vi "EVT Camera Get Value Enum Param.vi"(9 "value":u32, 10 "name":string, 11 "camera":u64) -> (1 "value out":u32, 3 "function return":u32(ring))   [LabVIEW 2019, in "EmergentCameraC.lvlib"]
doc: "EMERGENTCAMERAC_API EVT_ERROR EVT_CameraGetValueEnumParam(Camera_Handle camera, const char* name, unsigned int* value);"
uses:
  EmergentCameraC.lvlib
  emergentInstall_Windows/win64/eSDK/bin/EmergentCameraC.dll
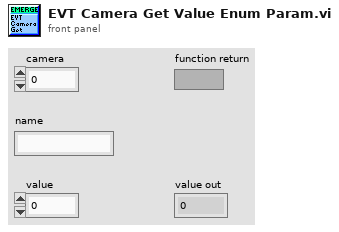
[diagram p1: front panel]
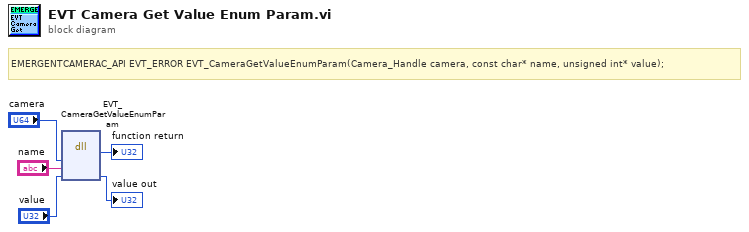
[diagram p0: block diagram]
diagram:
  # "EMERGENTCAMERAC_API EVT_ERROR EVT_CameraGetValueEnumParam(Camera_Handle camera, const char* name, unsigned int* value);"
  n1 = dll-call lib="E:/emergent/host-new_QT/emergentInstall_Windows/win64/eSDK/bin/EmergentCameraC.*" fn="EVT_CameraGetValueEnumParam"("camera"="camera", "name"="name", "value"="value") -> (→"function return":u32, "value"=→"value out":u32)  [unwired: 5 in, 2 out]
